vi "collect dataset.vi"() -> ()   [LabVIEW 2015]
uses:
  <vilib>/userdefined/High Color/IMAQdx.ctl
  <vilib>/Utility/file.llb/Write Delimited Spreadsheet (DBL).vi
  <vilib>/vision/driver/NI_Vision_Acquisition_Software.lvlib
  <resource>/objmgr/imaqdx.rc
panel:
  in  "save dataset":bool
  in  "File Name":path=path "C:/Documents and Settings/husmith/Desktop/CSVdata.csv"
  in  "camera mode":bool
  in  "base":i32(slide) scale=-125.0..125.0
  out "size(s)":i32
  in  "next photo":bool
  out "cy":dbl[](array[numeric])
  out "cx":dbl[](array[numeric])
  out "Image":T1(plugin-control)
  out "Circles":cluster{"x":dbl, "y":dbl, "r":dbl}[](array[cluster])
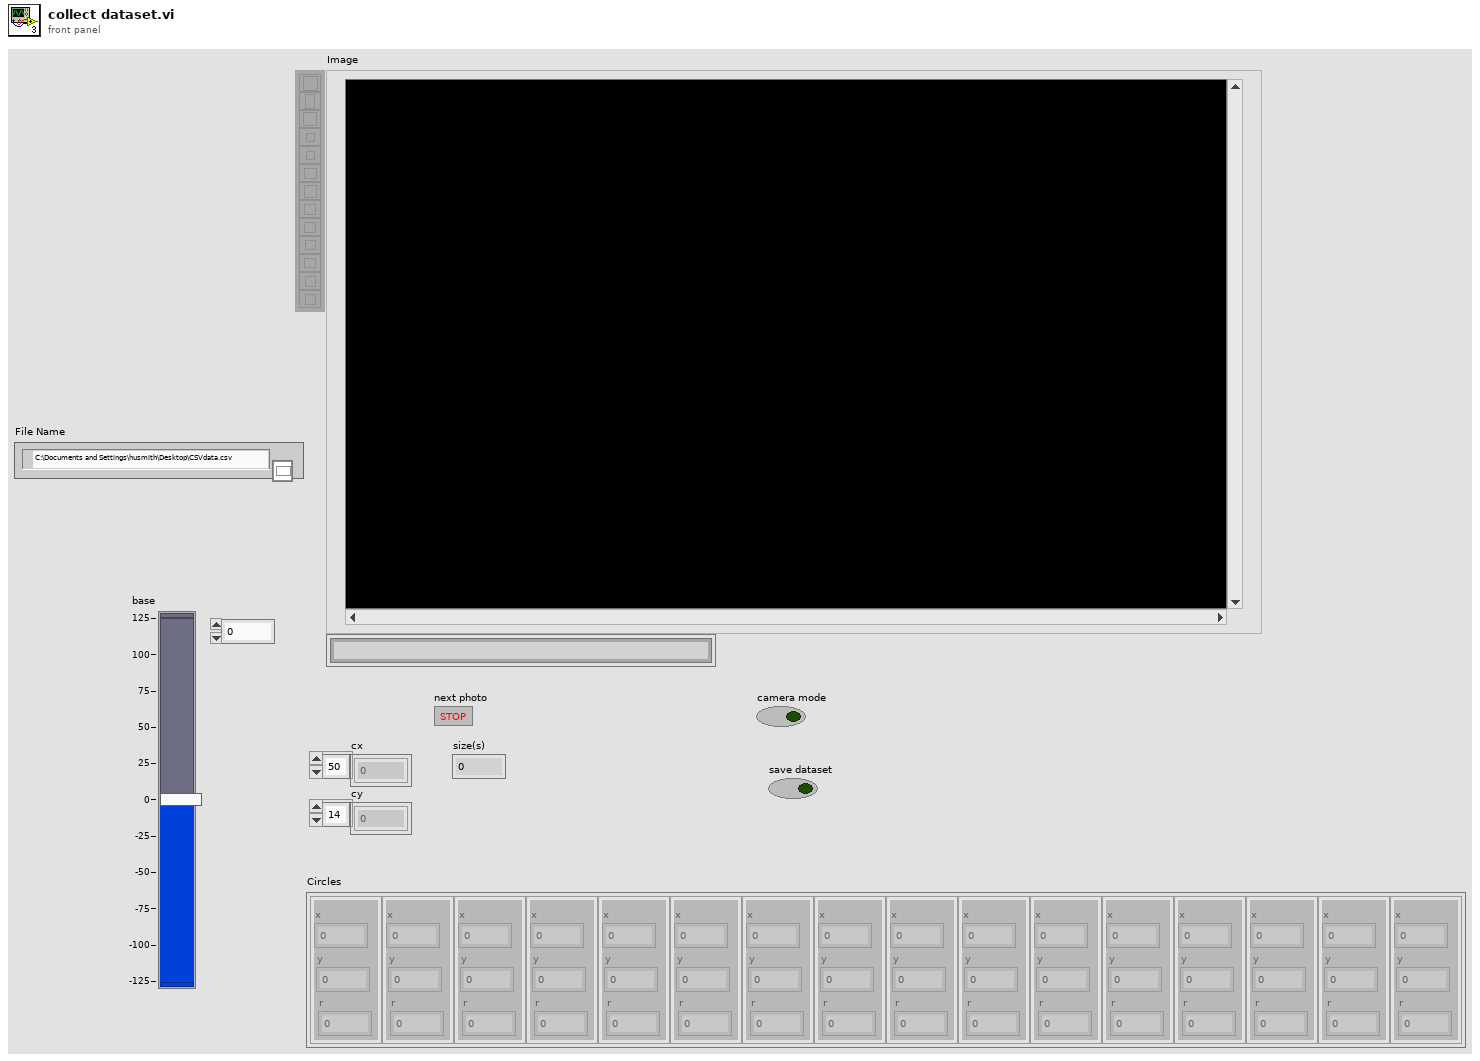
[diagram p1: front panel]
types:
  T1 = typedef "IMAQ Image.ctl" = refnum<image>
  T2 = typedef "IMAQdx.ctl" = refnum<k21>
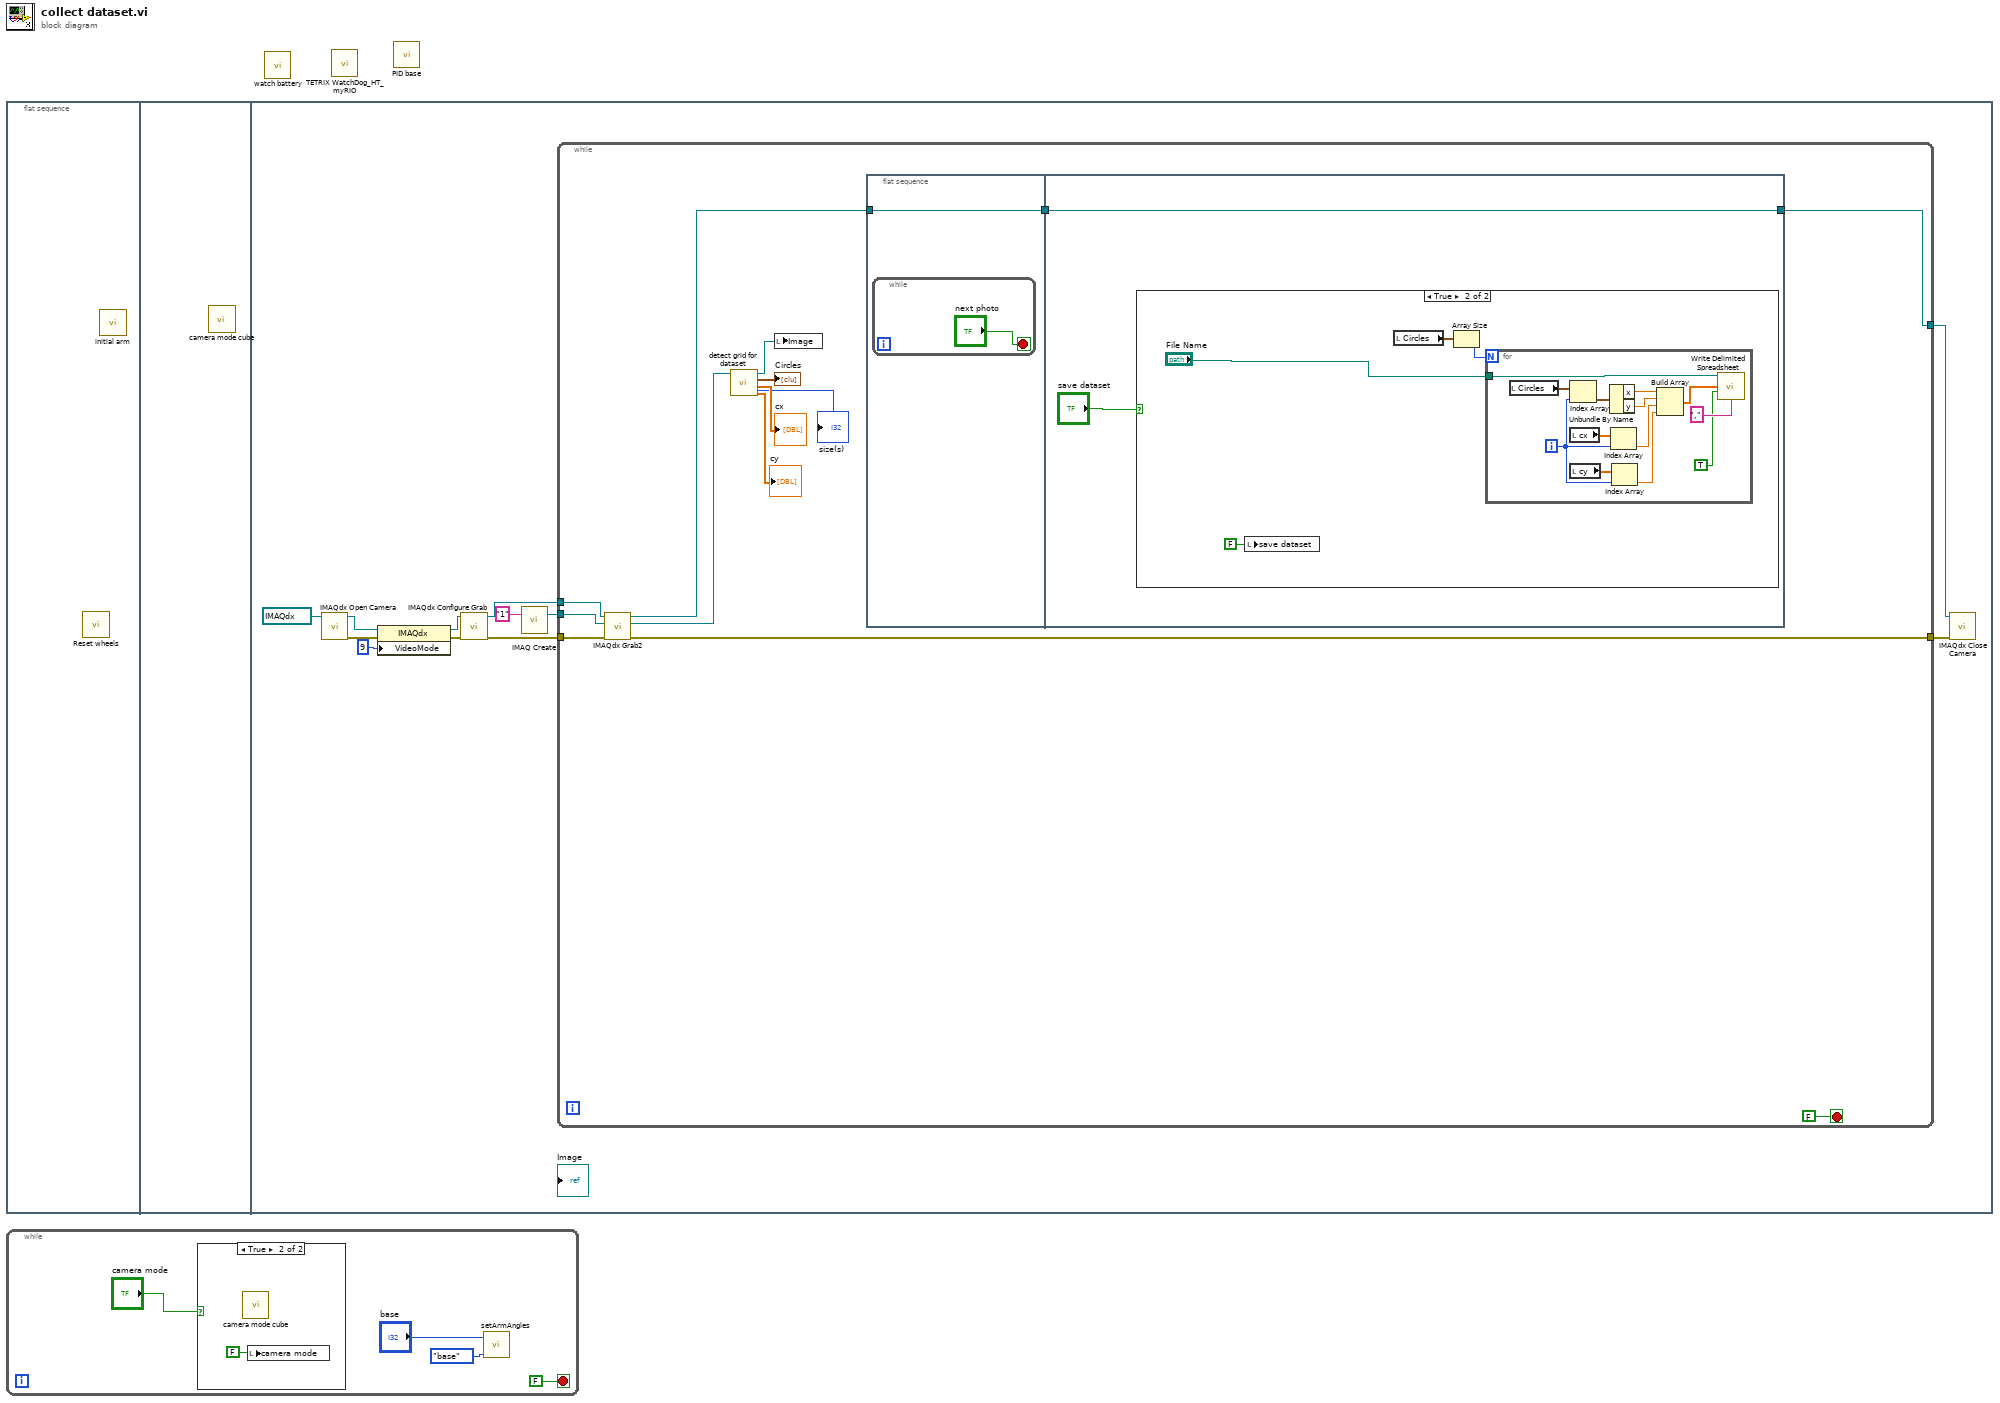
[diagram p0: block diagram]
diagram:
  n1 = flat-sequence {
    frame #0 {
      n2 = call "Reset wheels.vi"() -> ()  [unwired: 12 in]
      n3 = call "initial arm.vi"() -> ()  [unwired: 12 in]
    }
    frame #1 {
      n4 = call "camera mode cube.vi"() -> ()  [unwired: 12 in]
    }
    frame #2 {
      n5 = call <vilib>:"IMAQdx Open Camera.vi"("Session In"=T2 "cam0") -> ("error out"=w4:errorcluster, "Session Out"=w5:T2)  [unwired: 9 in]
      n6 = property class="IMAQdx"(reference=w5, error in=w4, "VideoMode"=u32 9) -> (reference out=w2:T2, error out=w3:errorcluster)
      n7 = call <vilib>:"IMAQdx Configure Grab.vi"("error in"=w3, "Session In"=w2) -> ("error out"=w11:errorcluster, "Session Out"=w10:T2)  [unwired: 8 in]
      n8 = call "IMAQ Create"("Image Name"="1") -> ("New Image"=w8:T1)  [unwired: 4 in, 1 out]
      n9 = while {
        tunnel: w11 -> [w26]
        tunnel: w10 -> [w25]
        tunnel: [w15] -> w9
        tunnel: w8 -> [w24]
        tunnel: [w23] -> w6
        stop <- FALSE stop-if-true
        n10 = call <vilib>:"IMAQdx Grab2.vi"("error in"=w26, "Image In"=w24, "Session In"=w25) -> ("error out"=w23:errorcluster, "Image Out"=w22:T1, "Session Out"=w14:T2)  [unwired: 5 in, 1 out]
        n11 = call "detect grid for dataset.vi"("Image 3"=w22) -> ("cy"=→"cy":dbl[], "cx"=→"cx":dbl[], "Circles"=→"Circles":cluster{"x":dbl, "y":dbl, "r":dbl}[], "Image 4"=w20:T1, "size(s)"=→"size(s)":i32)  [unwired: 6 in]
        n12 = local write "Image"(w20) -> ()
        n13 = flat-sequence {
          tunnel: w14 -> [w27]
          tunnel: [w27] -> w13
          tunnel: [w30] -> w15
          tunnel: w13 -> [w30]
          frame #0 {
            n14 = while {
              stop <- "next photo" stop-if-true
            }
          }
          frame #1 {
            n15 = case shown="True" "save dataset" {
              frame False {
              }
              frame True {
                n16 = local write "save dataset"(FALSE ("save dataset")) -> ()
                n17 = local read "Circles"() -> (w34:cluster{"x":dbl, "y":dbl, "r":dbl}[])
                n18 = Array Size(array=w34) -> (size(s)=w33:i32)
                n19 = for {
                  N: w33 -> [_]
                  tunnel: "File Name" -> [w36]
                  i -> [w44]
                  n20 = local read "Circles"() -> (w46:cluster{"x":dbl, "y":dbl, "r":dbl}[])
                  n21 = Index Array(array=w46, index=w44) -> (element=w45:cluster{"x":dbl, "y":dbl, "r":dbl})
                  n22 = local read "cx"() -> (w43:dbl[])
                  n23 = local read "cy"() -> (w42:dbl[])
                  n24 = Unbundle By Name(w45) -> ("x"=w41:dbl, "y"=w40:dbl)
                  n25 = Index Array(array=w43, index=w44) -> (element=w39:dbl)
                  n26 = Index Array(array=w42, index=w44) -> (element=w38:dbl)
                  n27 = Build Array(w41, w40, w39, w38) -> (w37:dbl[])
                  n28 = call-poly <vilib>:"Write Delimited Spreadsheet.vi"("file path (dialog if empty)"=w36, "1D data"=w37, "append to file? (F)"=TRUE ("append to file? (new file:F)"), "delimiter (\\t)"="," ("delimiter (\\t)")) -> ()  [unwired: 10 in, 2 out]
                }
              }
            }
          }
        }
      }
      n29 = call <vilib>:"IMAQdx Close Camera.vi"("error in"=w6, "Session In"=w9) -> ()  [unwired: 9 in, 1 out]
    }
  }
  n30 = while {
    stop <- FALSE stop-if-true
    n31 = case shown="True" "camera mode" {
      frame False {
      }
      frame True {
        n32 = call "camera mode cube.vi"() -> ()  [unwired: 12 in]
        n33 = local write "camera mode"(FALSE ("camera mode")) -> ()
      }
    }
    n34 = call "setArmAngles.vi"("Enum"=enum16{"shoulder", "elbow", "wrist", "base"}."base", "angle"="base") -> ()  [unwired: 2 in]
  }
  n35 = call "watch battery.vi"() -> ()  [unwired: 12 in]
  n36 = call <vilib>:"TETRIX WatchDog_HT_myRIO.vi"() -> ()  [unwired: 3 in, 1 out]
  n37 = call "PID base.vi"() -> ()  [unwired: 12 in]
